vi "Update Indicators (Data String to ref array).vi"(4 "Data String":string, 5 "Array":refnum<vi>[](array[refnum])) -> ()   [LabVIEW 2013]
panel:
  out "array":string[][](array[string])
  out "subarray":string[](array[string])
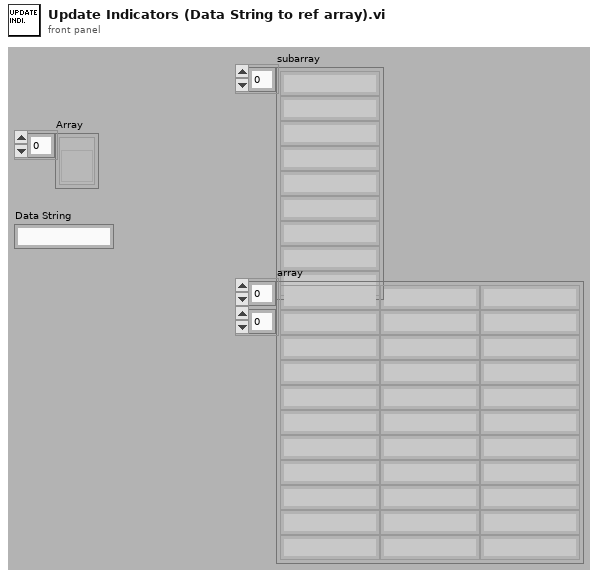
[diagram p1: front panel]
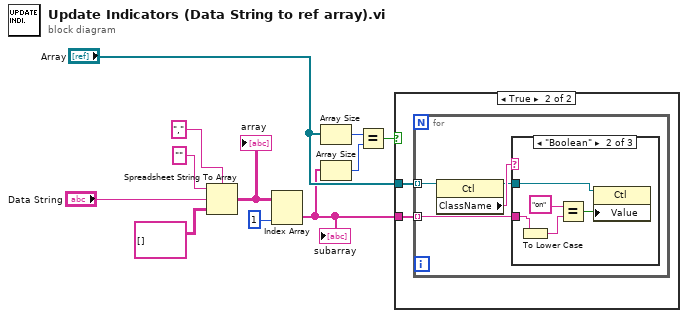
[diagram p0: block diagram]
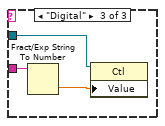
[diagram p4: hidden frame]
diagram:
  n1 = Spreadsheet String To Array(delimiter (Tab)=",", format string="", spreadsheet string="Data String", array type (2D Dbl)=string[][] []) -> (array=w4:string[][])
  "array" <- w4
  n2 = Index Array(array=w4, index (col)=1 ("disabled index (col)")) -> (element=w1:string[])  [unwired: 1 in]
  "subarray" <- w1
  n3 = Array Size(array="Array") -> (size(s)=w5:i32)
  n4 = Array Size(array=w1) -> (size(s)=w6:i32)
  n5 = Equal?(x=w5, y=w6) -> (x = y?=w2:bool)
  n6 = case shown="True" w2 {
    tunnel: "Array" -> [_ w13]
    tunnel: w1 -> [_ w12]
    frame False {
    }
    frame True {
      n7 = for {
        tunnel: w13 -> [w17] mode=indexing
        tunnel: w12 -> [w15] mode=indexing
        n8 = property class="Ctl"(reference=w17) -> (reference out=w14:refnum<vi>, "ClassName"=w16:string)  [unwired: 1 in, 1 out]
        n9 = case shown="\"Boolean\"" w16 {
          tunnel: w15 -> [_ w19 w23]
          tunnel: w14 -> [_ w21 w24]
          frame "False", Default {
          }
          frame "Boolean" {
            n10 = To Lower Case(string=w19) -> (all lower case string=w18:string)
            n11 = Equal?(x="on", y=w18) -> (x = y?=w20:bool)
            n12 = property class="Ctl"(reference=w21, "Value"=w20) -> ()  [unwired: 1 in, 2 out]
          }
          frame "Digital" {
            n13 = Fract/Exp String To Number(string=w23) -> (number=w25:dbl)  [unwired: 3 in, 1 out]
            n14 = property class="Ctl"(reference=w24, "Value"=w25) -> ()  [unwired: 1 in, 2 out]
          }
        }
      }
    }
  }
